vi "Get Screen Dimensions.vi"() -> (2 "screenWidth":i32, 3 "screenHeight":i32)   [LabVIEW 2015]
uses:
  user32.dll
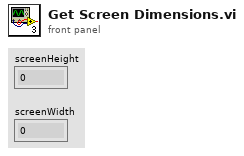
[diagram p1: front panel]
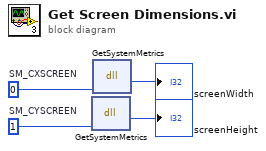
[diagram p0: block diagram]
diagram:
  w2 = 1  # SM_CYSCREEN
  w1 = 0  # SM_CXSCREEN
  n1 = dll-call lib="USER32.DLL" fn="GetSystemMetrics"("parameter"=w2) -> ("screenHeight"=→"screenHeight":i32)  [unwired: 4 in, 2 out]
  n2 = dll-call lib="USER32.DLL" fn="GetSystemMetrics"("parameter"=w1) -> ("screenWidth"=→"screenWidth":i32)  [unwired: 4 in, 2 out]
